vi "user process.vi"(8 "error in":errorcluster, 10 "Model State In":T1, 11 "Parameters to process":T3) -> (0 "error out":errorcluster, 2 "Model State Out":T1, 3 "Results from processing":T2)   [LabVIEW 2015, in "Temperature Chamber Model runtime.lvclass"]
uses:
  Temperature Chamber Model runtime.lvclass
  parameter user data.ctl
  result user data.ctl
  model state.ctl
  <vilib>/ptbypt/NI_PtbyPt.lvlib
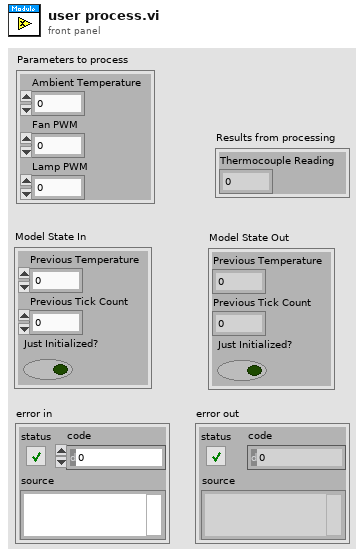
[diagram p1: front panel]
types:
  T1 = typedef "Temperature Chamber Model runtime.lvclass/model state.ctl" = cluster{"Previous Temperature":dbl, "Previous Tick Count":u32, "Just Initialized?":bool}
  T2 = typedef "Temperature Chamber Model runtime.lvclass/result user data.ctl" = cluster{"Thermocouple Reading":dbl}
  T3 = typedef "Temperature Chamber Model runtime.lvclass/parameter user data.ctl" = cluster{"Ambient Temperature":dbl, "Fan PWM":dbl, "Lamp PWM":dbl}
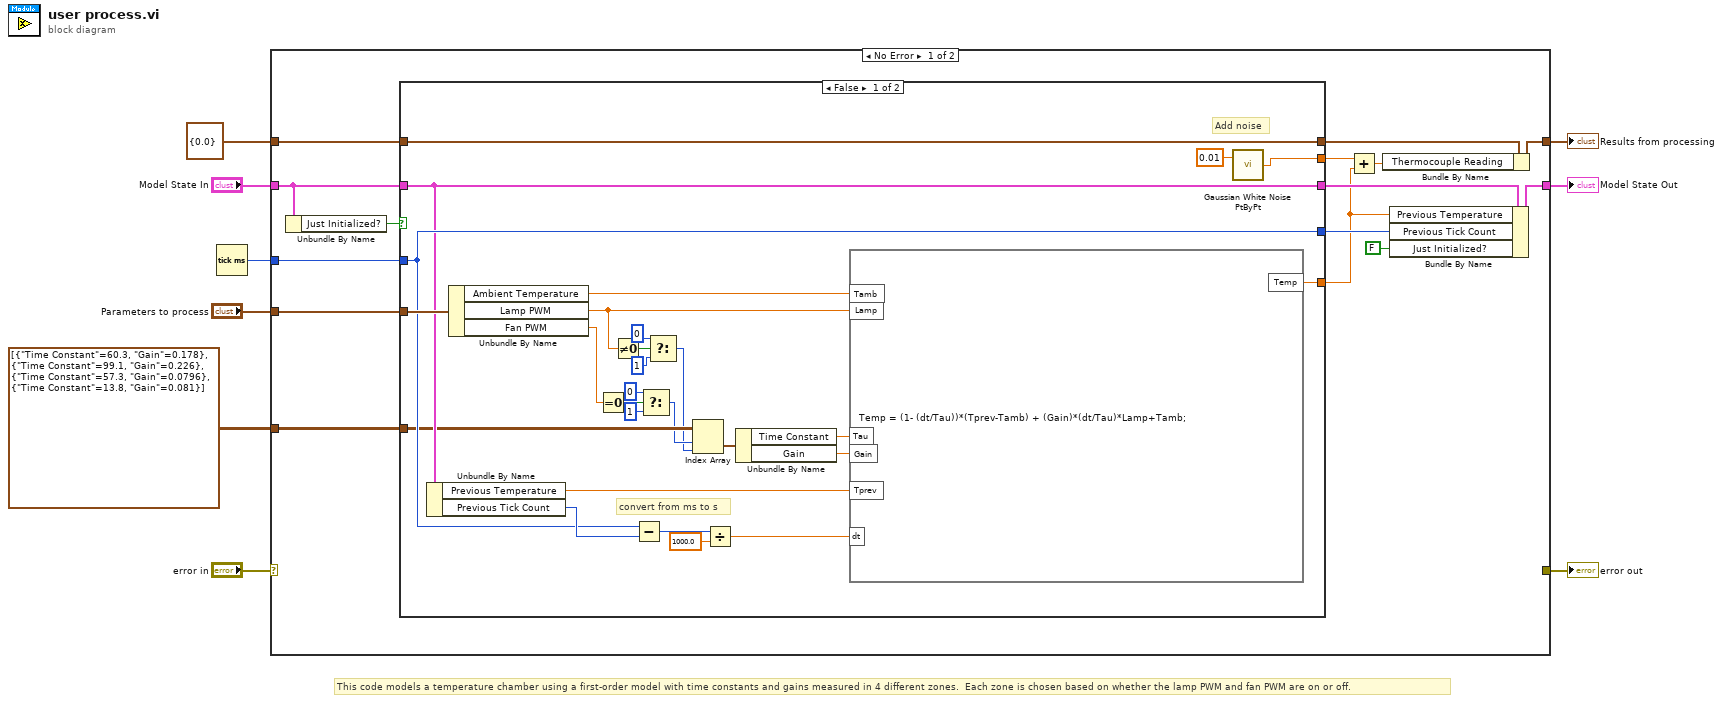
[diagram p0: block diagram]
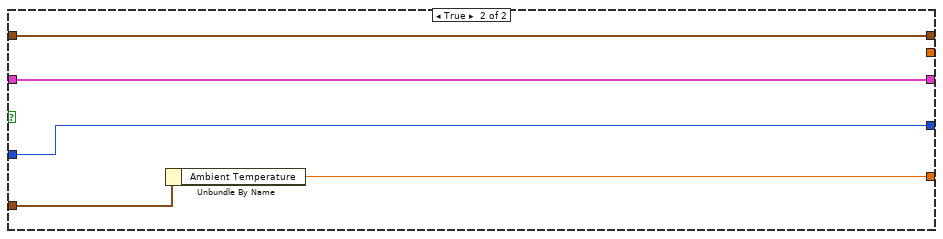
[diagram p2: hidden frame]
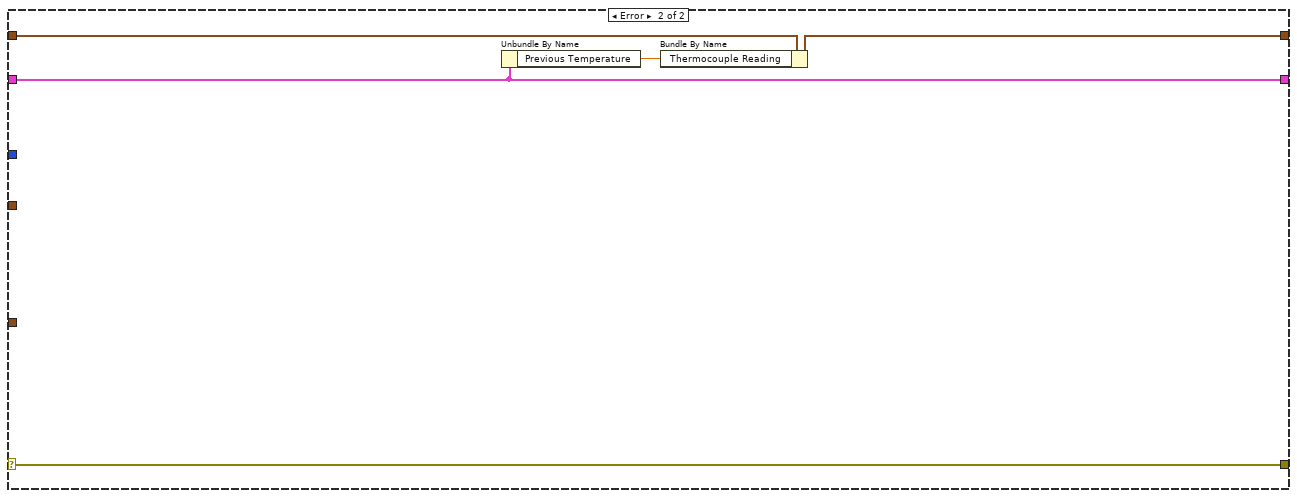
[diagram p3: hidden frame]
diagram:
  # "This code models a temperature chamber using a first-order model with time constants and gains measured in 4 different zones.  Each zone is chosen based on whether the lamp PWM and fan PWM are on or off."
  n1 = Tick Count (ms)() -> (millisecond timer value=w5:u32)
  n2 = case shown="No Error" "error in" {
    selector: "error in" -> [_ w61]
    tunnel: "Model State In" -> [w17 w58]
    tunnel: "Parameters to process" -> [w23 _]
    tunnel: [_ w61] -> w6
    tunnel: w5 -> [w18 _]
    tunnel: [w19 w58] -> w4
    tunnel: T2 {"Thermocouple Reading"=0.0} ("Results from processing") -> [w16 w60]
    tunnel: [w14 w59] -> w2
    tunnel: cluster{"Time Constant":dbl, "Gain":dbl}[][] [[{"Time Constant"=60.3, "Gain"=0.178}, {"Time Constant"=99.1, "Gain"=0.226}], [{"Time Constant"=57.3, "Gain"=0.0796}, {"Time Constant"=13.8, "Gain"=0.081}]] -> [w13 _]
    frame No Error {
      n3 = Unbundle By Name(w17) -> ("Just Initialized?"=w24:bool)
      n4 = case shown="False" w24 {
        tunnel: w23 -> [w51 w56]
        tunnel: [w41 w54] -> w22
        tunnel: [w42 w55] -> w12
        tunnel: [w48 w52] -> w21
        tunnel: w18 -> [w48 w52]
        tunnel: w17 -> [w41 w54]
        tunnel: w16 -> [w44 w53]
        tunnel: [w44 w53] -> w15
        tunnel: w13 -> [w40 _]
        tunnel: [w25 _] -> w11
        frame False {
          # "Add noise"
          # "convert from ms to s"
          n5 = Unbundle By Name(w41) -> ("Previous Temperature"=w50:dbl, "Previous Tick Count"=w49:u32)
          n6 = Unbundle By Name(w51) -> ("Ambient Temperature"=w43:dbl, "Lamp PWM"=w33:dbl, "Fan PWM"=w38:dbl)
          n7 = Equal To 0?(x=w38) -> (x = 0?=w37:bool)
          n8 = Not Equal To 0?(x=w33) -> (x != 0?=w30:bool)
          n9 = Subtract(x=w48, y=w49) -> (x-y=w46:u32)
          n10 = Select(t=u32 0, s=w37, f=u32 1) -> (s? t:f=w34:u32)
          n11 = Select(t=u32 0, s=w30, f=u32 1) -> (s? t:f=w29:u32)
          n12 = Index Array(array=w40, index (row)=w34, index (col)=w29) -> (element=w39:cluster{"Time Constant":dbl, "Gain":dbl})
          n13 = Divide(x=w46, y=1000.0) -> (x/y=w45:dbl)
          n14 = Unbundle By Name(w39) -> ("Time Constant"=w27:dbl, "Gain"=w28:dbl)
          n15 = formula code="Temp = (1- (dt/Tau))*(Tprev-Tamb) + (Gain)*(dt/Tau)*Lamp+Tamb;"("dt"=w45, "Tau"=w27, "Tprev"=w50, "Lamp"=w33, "Tamb"=w43, "Gain"=w28) -> ("Temp"=w42:dbl)
          n16 = call <vilib>:"Gaussian White Noise PtByPt.vi"("standard deviation"=0.01) -> ("Gaussian white noise"=w25:dbl)  [unwired: 2 in]
        }
        frame True {
          n17 = Unbundle By Name(w56) -> ("Ambient Temperature"=w55:dbl)
        }
      }
      n18 = Add(x=w11, y=w12) -> (x+y=w10:dbl)
      n19 = Bundle By Name(cluster=w15, "Thermocouple Reading"=w10) -> (w14:T2)
      n20 = Bundle By Name(cluster=w22, "Previous Temperature"=w12, "Previous Tick Count"=w21, "Just Initialized?"=FALSE) -> (w19:T1)
    }
    frame Error {
      n21 = Unbundle By Name(w58) -> ("Previous Temperature"=w57:dbl)
      n22 = Bundle By Name(cluster=w60, "Thermocouple Reading"=w57) -> (w59:T2)
    }
  }
  "error out" <- w6
  "Results from processing" <- w2
  "Model State Out" <- w4
